vi "XY Graph Shift Interpolated Plot.vi"(8 "Error In":errorcluster, 9 "Plot Interpolation (out)":T1, 10 "Plot Interpolation (in)":T1, 11 "Plot in":cluster{"t Array":dbl[], "Residual Array":dbl[]}) -> (0 "Error Out":errorcluster, 3 "Plot out":cluster{"t Array":dbl[], "Residual Array":dbl[]})   [LabVIEW 2021, in "AlliGator Decay Fit.lvlib"]
uses:
  AlliGator/Decay Analysis/Decay Fit/AlliGator Decay Fit.lvlib
  b0131b92-c6ea-47e1-9263-b06d56bd5151.vi
  LabVIEW Plot Interpolation.ctl
  Graphs.lvlib
panel:
  # "see the License on the block diagram (Ctrl+E or Window:Show Block Diagram)"
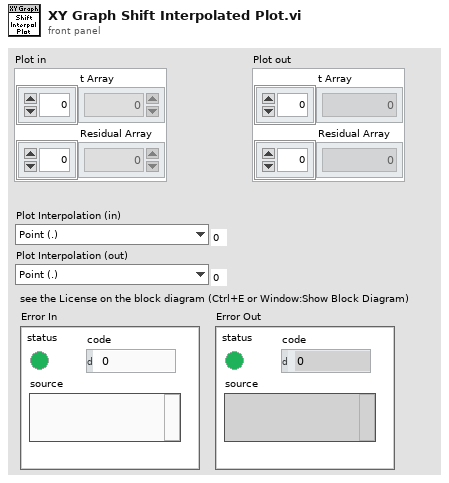
[diagram p1: front panel]
types:
  T1 = typedef "Graphs.lvlib/LabVIEW Plot Interpolation.ctl" = enum16{"Point (.)", "Stepwise Right (--.)", "Line + Point (\\. /)", "Stepwise Left (.--)", "Stepwise Centered (-.-)", "Stepwise Vertical (|.|)", "Line (-)", "Use Previous Plot's Style"}
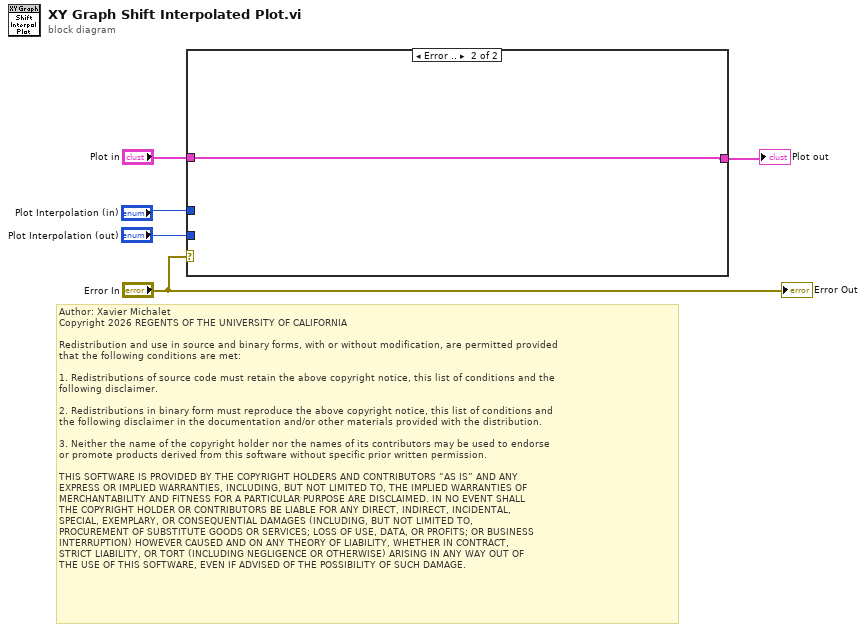
[diagram p0: block diagram]
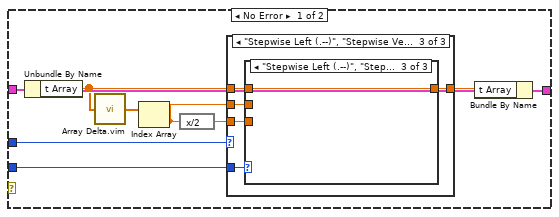
[diagram p2: hidden frame]
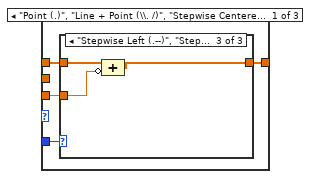
[diagram p3: hidden frame]
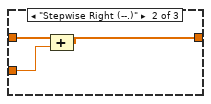
[diagram p5: hidden frame]
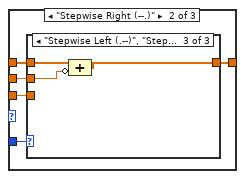
[diagram p6: hidden frame]
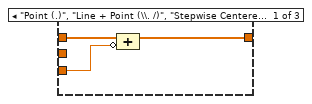
[diagram p7: hidden frame]
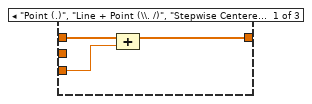
[diagram p9: hidden frame]
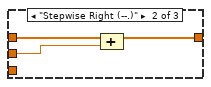
[diagram p10: hidden frame]
diagram:
  # "Author: Xavier Michalet\nCopyright 2026 REGENTS OF THE UNIVERSITY OF CALIFORNIA\n\nRedistribution and use in source and binary forms, with or without modification, are permitted provided\nthat the following conditions are met:\n\n1. Redistributions of source code must retain the above copyright notice, this list of conditions and the\nfollowing disclaimer.\n\n2. Redistributions in binary form must reproduce the above copyright notice, this list of conditions and\nthe following disclaimer in the documentation and/or other materials provided with the distribution.\n\n3. Neither the name of the copyright holder nor the names of its contributors may be used to endorse \nor promote products derived from this software without specific prior written permission.\n\nTHIS SOFTWARE IS PROVIDED BY THE COPYRIGHT HOLDERS AND CONTRIBUTORS “AS IS” AND ANY \nEXPRESS OR IMPLIED WARRANTIES, INCLUDING, BUT NOT LIMITED TO, THE IMPLIED WARRANTIES OF\nMERCHANTABILITY AND FITNESS FOR A PARTICULAR PURPOSE ARE DISCLAIMED. IN NO EVENT SHALL\nTHE COPYRIGHT HOLDER OR CONTRIBUTORS BE LIABLE FOR ANY DIRECT, INDIRECT, INCIDENTAL, \nSPECIAL, EXEMPLARY, OR CONSEQUENTIAL DAMAGES (INCLUDING, BUT NOT LIMITED TO, \nPROCUREMENT OF SUBSTITUTE GOODS OR SERVICES; LOSS OF USE, DATA, OR PROFITS; OR BUSINESS\nINTERRUPTION) HOWEVER CAUSED AND ON ANY THEORY OF LIABILITY, WHETHER IN CONTRACT, \nSTRICT LIABILITY, OR TORT (INCLUDING NEGLIGENCE OR OTHERWISE) ARISING IN ANY WAY OUT OF\nTHE USE OF THIS SOFTWARE, EVEN IF ADVISED OF THE POSSIBILITY OF SUCH DAMAGE."
  n1 = case shown="Error .." "Error In" {
    tunnel: "Plot in" -> [w14 w50]
    tunnel: [w13 w50] -> w4
    tunnel: "Plot Interpolation (in)" -> [w12 _]
    tunnel: "Plot Interpolation (out)" -> [w11 _]
    frame No Error {
      n2 = Unbundle By Name(w14) -> ("t Array"=w9:dbl[])
      n3 = call "Array Delta.vim"("A"=w9) -> ("A[i+1]-A[i]"=w8:dbl[])  [unwired: 8 in]
      n4 = Index Array(array=w8) -> (element=w6:dbl)  [unwired: 1 in]
      n5 = expression code="x/2"(w6) -> (w7:dbl)
      n6 = case shown="\"Stepwise Left (.--)\", \"Stepwise Vertical (|.|)\"" w12 {
        tunnel: w9 -> [w17 w29 w41]
        tunnel: w11 -> [w18 w30 w42]
        tunnel: [w16 w28 w40] -> w10
        tunnel: w7 -> [w15 w27 w39]
        tunnel: w6 -> [_ w26 w38]
        frame "Point (.)", "Line + Point (\\. /)", "Stepwise Centered (-.-)", "Line (-)", Default {
          n7 = case shown="\"Stepwise Left (.--)\", \"Stepwise Vertical (|.|)\"" w18 {
            tunnel: w17 -> [w19 w22 w25]
            tunnel: [w19 w20 w23] -> w16
            tunnel: w15 -> [_ w21 w24]
            frame "Point (.)", "Line + Point (\\. /)", "Stepwise Centered (-.-)", "Line (-)", Default {
            }
            frame "Stepwise Right (--.)" {
              n8 = Compound Arithmetic op=ADD(w22, w21) -> (w20:dbl[])
            }
            frame "Stepwise Left (.--)", "Stepwise Vertical (|.|)" {
              n9 = Compound Arithmetic op=ADD(w25, invert w24) -> (w23:dbl[])
            }
          }
        }
        frame "Stepwise Right (--.)" {
          n10 = case shown="\"Stepwise Left (.--)\", \"Stepwise Vertical (|.|)\"" w30 {
            tunnel: w29 -> [w33 w34 w37]
            tunnel: [w32 w34 w36] -> w28
            tunnel: w27 -> [w31 _ _]
            tunnel: w26 -> [_ _ w35]
            frame "Point (.)", "Line + Point (\\. /)", "Stepwise Centered (-.-)", "Line (-)", Default {
              n11 = Compound Arithmetic op=ADD(w33, invert w31) -> (w32:dbl[])
            }
            frame "Stepwise Right (--.)" {
            }
            frame "Stepwise Left (.--)", "Stepwise Vertical (|.|)" {
              n12 = Compound Arithmetic op=ADD(w37, invert w35) -> (w36:dbl[])
            }
          }
        }
        frame "Stepwise Left (.--)", "Stepwise Vertical (|.|)" {
          n13 = case shown="\"Stepwise Left (.--)\", \"Stepwise Vertical (|.|)\"" w42 {
            tunnel: w41 -> [w45 w48 w49]
            tunnel: [w44 w47 w49] -> w40
            tunnel: w39 -> [w43 _ _]
            tunnel: w38 -> [_ w46 _]
            frame "Point (.)", "Line + Point (\\. /)", "Stepwise Centered (-.-)", "Line (-)", Default {
              n14 = Compound Arithmetic op=ADD(w45, w43) -> (w44:dbl[])
            }
            frame "Stepwise Right (--.)" {
              n15 = Compound Arithmetic op=ADD(w48, w46) -> (w47:dbl[])
            }
            frame "Stepwise Left (.--)", "Stepwise Vertical (|.|)" {
            }
          }
        }
      }
      n16 = Bundle By Name(cluster=w14, "t Array"=w10) -> (w13:cluster{"t Array":dbl[], "Residual Array":dbl[]})
    }
    frame Error {
    }
  }
  "Plot out" <- w4
  "Error Out" <- "Error In"
